vi "picture.get2.vi"(11 "midi-ui in":refnum<class "midi-ui.lvclass">) -> (2 "image":picture)   [LabVIEW 2020, in "midi-ui.lvclass"]
uses:
  midi-ui.lvclass
  midi-ui.lvclass/midi-ui.ctl
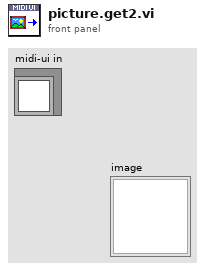
[diagram p1: front panel]
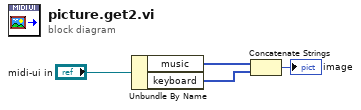
[diagram p0: block diagram]
diagram:
  n1 = Unbundle By Name("midi-ui in") -> ("music"=w3:picture[], "keyboard"=w4:picture[])
  n2 = Concatenate Strings(w3, w4) -> (→"image":picture)
